vi "pullNodeFromOpen.vi"(8 "error in (no error)":errorcluster, 11 "MultiTree in":refnum<class "MultiTree.lvclass">) -> (0 "error out":errorcluster, 1 "empty":bool, 2 "RemovedNode":refnum<data-value>, 3 "MultiTree out":refnum<class "MultiTree.lvclass">)   [LabVIEW 2014, in "MultiTree.lvlib" / "MultiTree.lvclass"]
uses:
  <userlib>/AdvancedDataStructures/ClassBased/MultiTree/MultiTree.lvclass
  <userlib>/AdvancedDataStructures/ClassBased/MultiTreeNode/MultiTreeNode.lvclass
  <userlib>/AdvancedDataStructures/ClassBased/MultiTree/MultiTree.lvclass/MultiTree.ctl
  <userlib>/AdvancedDataStructures/ClassBased/LinkedList/position.ctl
  <userlib>/AdvancedDataStructures/ClassBased/LinkedList/LinkedList.lvclass
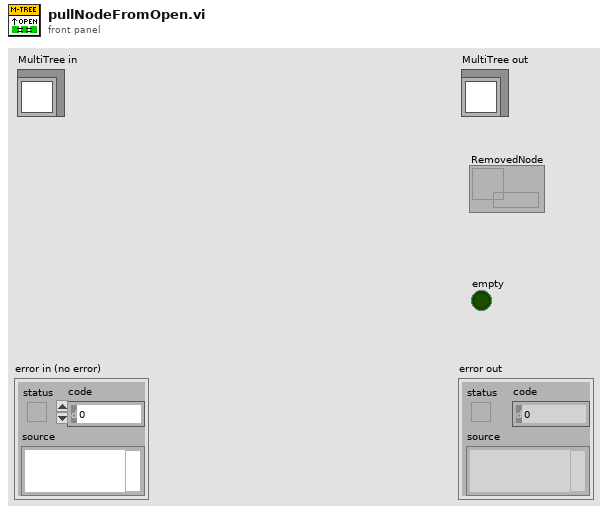
[diagram p1: front panel]
types:
  T1 = typedef "LinkedList.lvlib/LinkedList.lvclass/position.ctl" = enum16{"Front", "Back", "Search"}
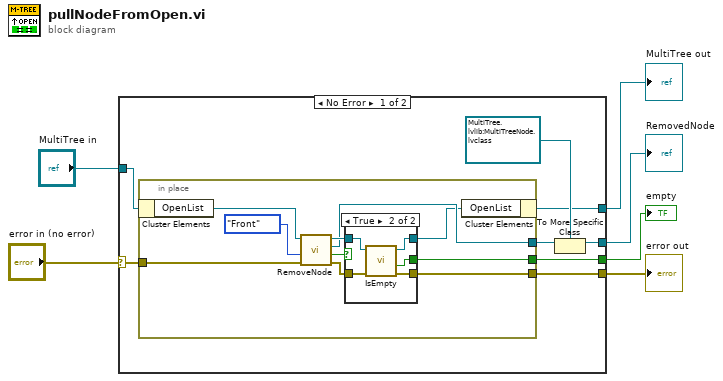
[diagram p0: block diagram]
diagram:
  n1 = case shown="No Error" "error in (no error)" {
    selector: "error in (no error)" -> [w12 w33]
    tunnel: [w9 w33] -> w5
    tunnel: [w10 w32] -> w3
    tunnel: "MultiTree in" -> [w11 w32]
    tunnel: [w8 _] -> w2
    tunnel: [w7 _] -> w1
    frame No Error {
      n2 = in-place {
        in-place-border: w12 -> [w23]
        in-place-border: [w18] -> w7
        in-place-border: [w17] -> w14
        in-place-border: [w15] -> w9
        n3 = in-place-cluster #1(w11) -> ("OpenList"=w24:refnum<class "BasicSortedList.lvclass">)
        n4 = call <userlib>:"RemoveNode.vi"("error in (no error)"=w23, "position"=position."Front", "LinkedList in"=w24) -> ("error out"=w19:errorcluster, "ignored"=w20:bool, "RemovedNode"=w17:refnum<data-value>, "LinkedList out"=w21:refnum<class "BasicSortedList.lvclass">)  [unwired: 5 in]
        n5 = case shown="True" w20 {
          tunnel: w21 -> [w26 w31]
          tunnel: w19 -> [w25 w30]
          tunnel: [_ w29] -> w18
          tunnel: [w26 w28] -> w16
          tunnel: [w25 w27] -> w15
          frame False {
          }
          frame True {
            n6 = call <userlib>:"IsEmpty.vi"("error in (no error)"=w30, "LinkedList in"=w31) -> ("error out"=w27:errorcluster, "empty"=w29:bool, "LinkedList out"=w28:refnum<class "BasicSortedList.lvclass">)  [unwired: 7 in]
          }
        }
        n7 = in-place-cluster #1("OpenList"=w16) -> (w10:refnum<class "MultiTree.lvclass">)
      }
      n8 = To More Specific Class(target class=refnum<data-value> refnum ("data value reference"), reference=w14) -> (specific class reference=w8:refnum<data-value>)  [unwired: 1 in, 1 out]
    }
    frame Error {
    }
  }
  "error out" <- w5
  "MultiTree out" <- w3
  "empty" <- w1
  "RemovedNode" <- w2
